vi "tm_getdcimgframe8_40.vi"(7 "Options":i32(ring) items=["no option"=0, "high contrast"=16], 8 "error in (no error)":errorcluster, 10 "Frame Index":i32=-1, 11 "File Handle in":u32) -> (0 "error out":errorcluster, 1 "Timestamp":dbl, 2 "Data":u8[][](array[numeric]), 3 "File Handle out":u32)   [LabVIEW 2011]
uses:
  tmcamcon.dll
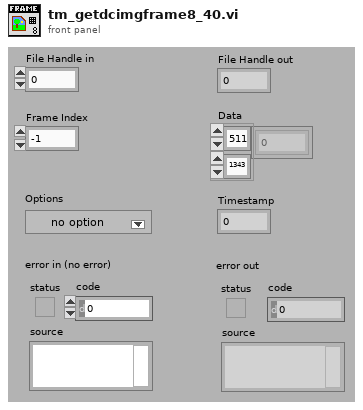
[diagram p1: front panel]
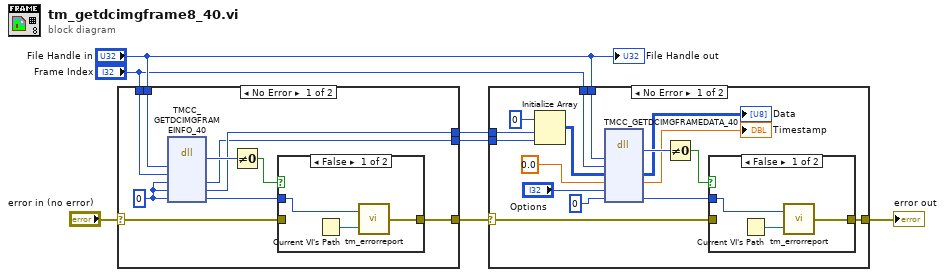
[diagram p0: block diagram]
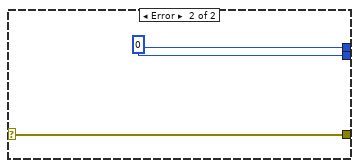
[diagram p5: hidden frame]
diagram:
  n1 = case shown="No Error" "error in (no error)" {
    selector: "error in (no error)" -> [w11 w23]
    tunnel: [w8 w23] -> w6
    tunnel: "File Handle in" -> [w16 _]
    tunnel: [w12 w22] -> w3
    tunnel: [w13 w22] -> w4
    tunnel: "Frame Index" -> [w14 _]
    frame No Error {
      w15 = 0 ("Erval")
      n2 = dll-call lib="tmcamcon.dll" fn="TMCC_GETDCIMGFRAMEINFO_40"("index"=w16, "frameindex"=w14, "width"=w15, "height"=w15, "Erval"=w15) -> ("return type"=w17:u32, "width"=w12:i32, "height"=w13:i32, "Erval"=w10:i32)  [unwired: 5 in, 2 out]
      n3 = Not Equal To 0?(x=w17) -> (x != 0?=w9:bool)
      n4 = case shown="False" w9 {
        tunnel: w11 -> [_ w21]
        tunnel: [w19 w21] -> w8
        tunnel: w10 -> [w18 _]
        frame False {
          n5 = Current VI's Path() -> (path=w20:path)
          n6 = call <userlib>:"tm_errorreport.vi"("Source"=w20, "Error"=w18) -> ("error out"=w19:errorcluster)
        }
        frame True {
        }
      }
    }
    frame Error {
      w22 = 0 ("buf")
    }
  }
  n7 = case shown="No Error" w6 {
    selector: w6 -> [w28 w44]
    tunnel: [w25 w44] -> w2
    tunnel: "File Handle in" -> [w38 _]
    tunnel: w4 -> [w36 _]
    tunnel: w3 -> [w35 _]
    tunnel: "Frame Index" -> [w32 _]
    frame No Error {
      n8 = Initialize Array(u8 0 ("buf"), w36, w35) -> (w34:u8[][])
      n9 = dll-call lib="tmcamcon.dll" fn="TMCC_GETDCIMGFRAMEDATA_40"("index"=w38, "frame"=w32, "imgarray"=w34, "timestamp"=0.0 ("Erval"), "option"="Options", "Erval"=0) -> ("return type"=w39:u32, "imgarray"=→"Data":u8[][], "timestamp"=→"Timestamp":dbl, "Erval"=w27:i32)  [unwired: 6 in, 2 out]
      n10 = Not Equal To 0?(x=w39) -> (x != 0?=w26:bool)
      n11 = case shown="False" w26 {
        tunnel: w28 -> [_ w43]
        tunnel: [w41 w43] -> w25
        tunnel: w27 -> [w40 _]
        frame False {
          n12 = Current VI's Path() -> (path=w42:path)
          n13 = call <userlib>:"tm_errorreport.vi"("Source"=w42, "Error"=w40) -> ("error out"=w41:errorcluster)
        }
        frame True {
        }
      }
    }
    frame Error {
    }
  }
  "error out" <- w2
  "File Handle out" <- "File Handle in"
